vi "9239_conversions.vi"(11 "data":dbl[](array[numeric])) -> (3 "Array":dbl[](array[numeric]))   [LabVIEW 2019]
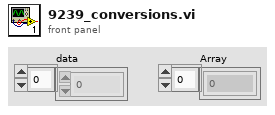
[diagram p1: front panel]
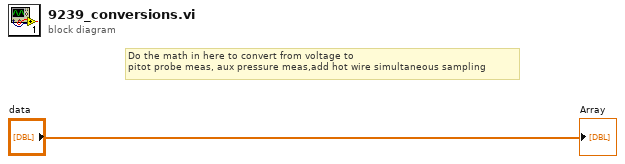
[diagram p0: block diagram]
diagram:
  # "Do the math in here to convert from voltage to \npitot probe meas, aux pressure meas,add hot wire simultaneous sampling"
  "Array" <- "data"
